vi "_Definition.vi"() -> (2 "Definition":T1)   [LabVIEW 2022 SP3, in "Conditum-Example.lvlib" / "Game.lvclass"]
uses:
  Game.lvclass
  Game.lvclass/Game.ctl
  Conditum/Relation Mapping.ctl
  Conditum/Conditum.lvlib
  Conditum/Entity/Entity.lvclass
  Conditum/Columns/Relation/Definition.ctl
  Conditum/Columns/Relation/Relation.lvclass
  Conditum/Columns/Type/Definition.ctl
  Conditum/Columns/Type/Type.lvclass
  Conditum/Columns/Relation/Relation Definition.ctl
  User/User.lvclass
  Conditum/Columns/String/Definition.ctl
  Conditum/Columns/String/String.lvclass
  Conditum/Attributes.ctl
  Conditum/Columns/String/String Definition.ctl
  Conditum/Columns/Timestamp/Timestamp.lvclass
  Conditum/Columns/Timestamp/Definition.ctl
  Conditum/Columns/Timestamp/DateTime Definition.ctl
  Conditum/Columns/Boolean/Boolean.lvclass
  Conditum/Columns/Boolean/Definition.ctl
  Conditum/Columns/Boolean/Boolean Definition.ctl
  Conditum/Columns/Entity/Entity.lvclass
  Conditum/Columns/Entity Collection/Entity Collection.lvclass
  C:/dev/lv/illuminated-g/lv-conditum/Conditum/Entity/Entity.lvclass
  C:/dev/lv/illuminated-g/lv-conditum/Conditum-Example/User/User.lvclass
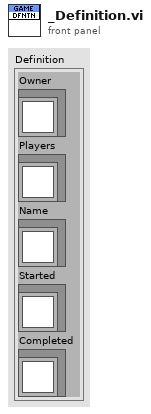
[diagram p1: front panel]
types:
  T1 = cluster{"Owner":refnum<class "Entity.lvclass">, "Players":refnum<class "Entity Collection.lvclass">, "Name":refnum<class "String.lvclass">, "Started":refnum<class "Timestamp.lvclass">, "Completed":refnum<class "Boolean.lvclass">}
  T2 = typedef "Conditum.lvlib/Columns.lvlib/Boolean.lvclass/Boolean Definition.ctl" = cluster{"Type":T3, "Attributes":T4, "Boolean":T5}
  T3 = typedef "Conditum.lvlib/Columns.lvlib/Type.lvclass/Definition.ctl" = cluster{"Table Name":string, "Nullable":bool, "Default NULL":bool}
  T4 = typedef "Conditum.lvlib/Attributes.ctl" = cluster{"Primary Key":bool, "Unique":bool, "Foreign Key":bool}
  T5 = typedef "Conditum.lvlib/Columns.lvlib/Boolean.lvclass/Definition.ctl" = cluster{"Default":bool}
  T6 = typedef "Conditum.lvlib/Columns.lvlib/Timestamp.lvclass/DateTime Definition.ctl" = cluster{"Type":T3, "Attributes":T4, "DateTime":T7}
  T7 = typedef "Conditum.lvlib/Columns.lvlib/Timestamp.lvclass/Definition.ctl" = cluster{"Default":timestamp}
  T8 = typedef "Conditum.lvlib/Columns.lvlib/Relation.lvclass/Relation Definition.ctl" = cluster{"Type":T3, "Relation":T9}
  T9 = typedef "Conditum.lvlib/Columns.lvlib/Relation.lvclass/Definition.ctl" = cluster{"Related To":refnum<class "Entity.lvclass">, "Mapping":T10, "Reversed By":string}
  T10 = typedef "Conditum.lvlib/Relation Mapping.ctl" = enum16{"OneToMany", "ManyToOne", "ManyToMany", "OneToOne"}
  T11 = typedef "Conditum.lvlib/Columns.lvlib/String.lvclass/String Definition.ctl" = cluster{"Type":T3, "Attributes":T4, "String":T12}
  T12 = typedef "Conditum.lvlib/Columns.lvlib/String.lvclass/Definition.ctl" = cluster{"Default":string, "Length":i32}
  T13 = cluster{"Entity out":refnum<class "Entity.lvclass">, "Entity Collection out":refnum<class "Entity Collection.lvclass">, "String out":refnum<class "String.lvclass">, "DateTime out":refnum<class "Timestamp.lvclass">, "Boolean out":refnum<class "Boolean.lvclass">}
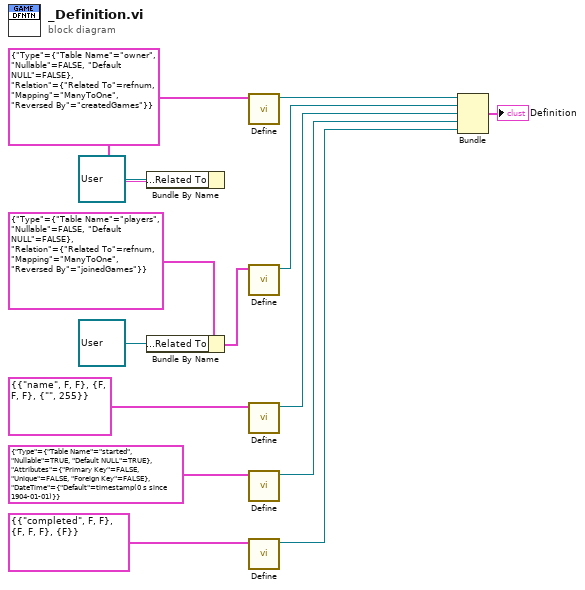
[diagram p0: block diagram]
diagram:
  w8 = T8 {"Type"={"Table Name"="owner", "Nullable"=FALSE, "Default NULL"=FALSE}, "Relation"={"Related To"=refnum, "Mapping"=enum."ManyToOne", "Reversed By"="createdGames"}} ("Relation Definition")
  n1 = Bundle By Name(cluster=w8, "Relation.Related To"=refnum<class "User.lvclass"> refnum ("Conditum-Example.lvlib:User.lvclass")) -> ()  [unwired: 1 out]
  n2 = Bundle By Name(cluster=T8 {"Type"={"Table Name"="players", "Nullable"=FALSE, "Default NULL"=FALSE}, "Relation"={"Related To"=refnum, "Mapping"=enum."ManyToOne", "Reversed By"="joinedGames"}} ("Relation Definition"), "Relation.Related To"=refnum<class "User.lvclass"> refnum ("Conditum-Example.lvlib:User.lvclass")) -> (w7:T8)
  n3 = call "Define.vi"("Relation Definition"=w8) -> ("Entity out"=w6:refnum<class "Entity.lvclass">)  [unwired: 10 in]
  n4 = call "Define.vi"("Relation Definition"=w7) -> ("Entity Collection out"=w5:refnum<class "Entity Collection.lvclass">)  [unwired: 10 in]
  n5 = call "Define.vi"("Definition"=T11 {"Type"={"Table Name"="name", "Nullable"=FALSE, "Default NULL"=FALSE}, "Attributes"={"Primary Key"=FALSE, "Unique"=FALSE, "Foreign Key"=FALSE}, "String"={"Default"="", "Length"=255}}) -> ("String out"=w4:refnum<class "String.lvclass">)  [unwired: 10 in]
  n6 = call "Define.vi"("Definition"=T6 {"Type"={"Table Name"="started", "Nullable"=TRUE, "Default NULL"=TRUE}, "Attributes"={"Primary Key"=FALSE, "Unique"=FALSE, "Foreign Key"=FALSE}, "DateTime"={"Default"=timestamp(0 s since 1904-01-01)}}) -> ("DateTime out"=w3:refnum<class "Timestamp.lvclass">)  [unwired: 10 in]
  n7 = call "Define.vi"("Init Data"=T2 {"Type"={"Table Name"="completed", "Nullable"=FALSE, "Default NULL"=FALSE}, "Attributes"={"Primary Key"=FALSE, "Unique"=FALSE, "Foreign Key"=FALSE}, "Boolean"={"Default"=FALSE}}) -> ("Boolean out"=w2:refnum<class "Boolean.lvclass">)  [unwired: 10 in]
  n8 = Bundle("Entity out"=w6, "Entity Collection out"=w5, "String out"=w4, "DateTime out"=w3, "Boolean out"=w2) -> (→"Definition":T13)  [unwired: 1 in]
